vi "Simulator ATT Version.vi"() -> ()   [LabVIEW 2011]
uses:
  Summitek EXT/Miscellaneous/OGAB Version.ctl
panel:
  in  "DriverType":string="ATT"
  in  "Version":T1={"Version"="6.3", "Build Number"=12, "Build Date/Time"=3440694548.419435} {"Build Date/Time" format="%<%X\n%x>T"}
  # "Note: The version\nglobal is set during\nbuild.  Don't change\nor rename this variable"
  # "The DriverType goes here -\nmake sure to \"Make Current\nValue Default\""
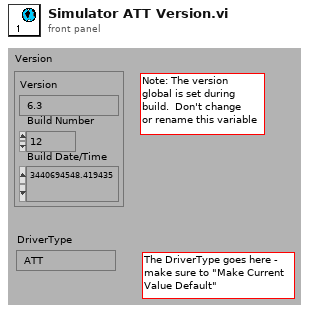
[diagram p1: front panel]
types:
  T1 = typedef "OGAB Version.ctl" = cluster{"Version":string, "Build Number":u32, "Build Date/Time":dbl}
diagram:
